vi "CMI ADS127L21 - Get Record Timestamp.vi"(8 "error in (no error)":errorcluster, 10 "Use binary mode? (False)":bool, 11 "session in":T1 {"channels"."Channel" min=1 max=8 step=1}) -> (0 "error out":errorcluster, 2 "timestamp [s]":ext, 3 "session out":T1 {"channels"."Channel" min=1 max=8 step=1})   [LabVIEW 2020]
doc: "Get timestamp of last record. USe of binary mode will transfer timestamp as int64 and then it is divided by sampling rate. This should overcome limited resolution of float64."
uses:
  CMI ADS127L21 - Session.ctl
  CMI ADS127L21 - Record Channel.ctl
  CMI ADS127L21 - Input Range.ctl
  CMI ADS127L21 - Input Mode.ctl
  CMI ADS127L21 - Input Impedance.ctl
  CMI ADS127L21 - EXTOUT Mode.ctl
  CMI ADS127L21 - EXTOUT Polarity.ctl
  <vilib>/Instr/_visa.llb/VISA Flush IO Buffer Mask.ctl
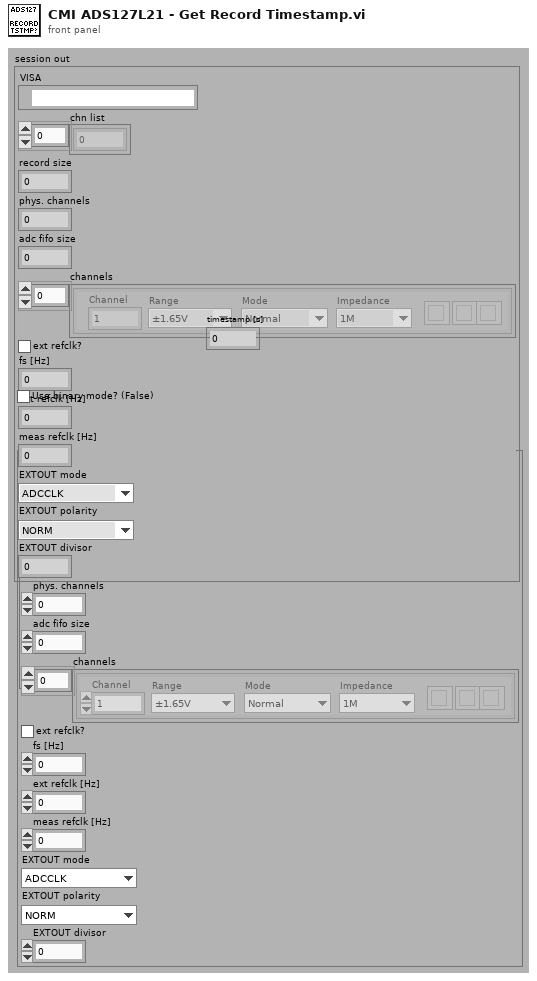
[diagram p1: front panel]
types:
  T1 = typedef "CMI ADS127L21 - Session.ctl" = cluster{"VISA":refnum<visa-resource-name>, "chn list":i32[], "record size":i32, "phys. channels":i32, "adc fifo size":i32, "channels":T2[], "ext refclk?":bool, "fs [Hz]":dbl, "ext refclk [Hz]":dbl, "meas refclk [Hz]":dbl, "EXTOUT mode":T6, "EXTOUT polarity":T7, "EXTOUT divisor":i32}
  T2 = typedef "CMI ADS127L21 - Record Channel.ctl" = cluster{"Range":T3, "Channel":i32, "Mode":T4, "Impedance":T5, "btn clr":bool, "btn up":bool, "btn down":bool}
  T3 = typedef "CMI ADS127L21 - Input Range.ctl" = enum16{"±1.65V", "±2V"}
  T4 = typedef "CMI ADS127L21 - Input Mode.ctl" = enum16{"Normal", "Inverted", "GND"}
  T5 = typedef "CMI ADS127L21 - Input Impedance.ctl" = enum16{"1M", "1k5"}
  T6 = typedef "CMI ADS127L21 - EXTOUT Mode.ctl" = enum16{"ADCCLK", "REFCLK", "SMPLCLK", "FIRST"}
  T7 = typedef "CMI ADS127L21 - EXTOUT Polarity.ctl" = enum16{"NORM", "INV"}
  T8 = typedef "VISA Flush IO Buffer Mask.ctl" = u16
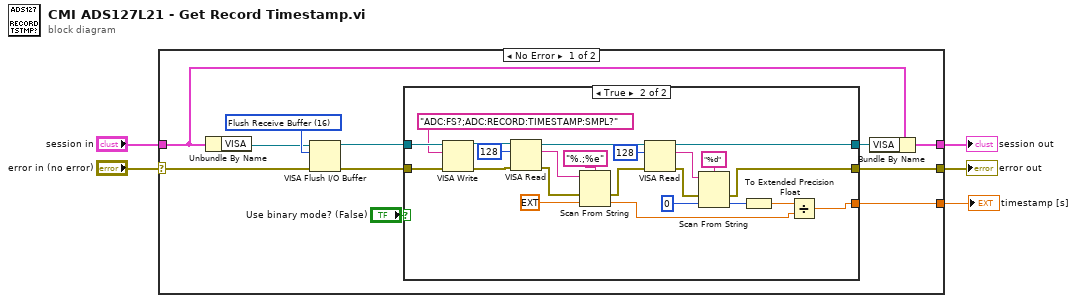
[diagram p0: block diagram]
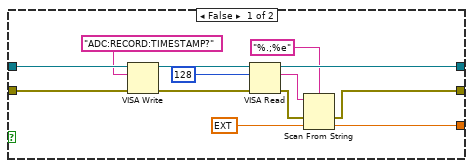
[diagram p2: hidden frame]
diagram:
  n1 = case shown="No Error" "error in (no error)" {
    selector: "error in (no error)" -> [w13 w54]
    tunnel: "session in" -> [w6 w53]
    tunnel: [w16 w53] -> w4
    tunnel: [w9 w54] -> w3
    tunnel: [w8 _] -> w1
    frame No Error {
      w15 = T8 16 items=["Flush Receive Buffer"=16, "Write Transmit Buffer to Device"=32, "Flush Receive Buffer (No I/O)"=64, "Flush Transmit Buffer"=128] ("Mask")
      n2 = Unbundle By Name(w6) -> ("VISA"=w14:refnum<visa-resource-name>)
      n3 = VISA Flush I/O Buffer(VISA resource name=w14, mask (16)=w15, error in (no error)=w13) -> (VISA resource name out=w11:refnum<visa-resource-name>, error out=w12:errorcluster)
      n4 = case shown="True" "Use binary mode? (False)" {
        tunnel: w12 -> [w29 w52]
        tunnel: w11 -> [w28 w51]
        tunnel: [w24 w49] -> w10
        tunnel: [w20 w46] -> w9
        tunnel: [w17 w41] -> w8
        frame False {
          n5 = VISA Write(VISA resource name=w28, write buffer="ADC:RECORD:TIMESTAMP?", error in (no error)=w29) -> (VISA resource name out=w25:refnum<visa-resource-name>, error out=w26:errorcluster)  [unwired: 1 out]
          n6 = VISA Read(VISA resource name=w25, byte count=u32 128, error in (no error)=w26) -> (VISA resource name out=w24:refnum<visa-resource-name>, read buffer=w21:string, error out=w22:errorcluster)  [unwired: 1 out]
          n7 = Scan From String(format string="%.;%e", input string=w21, error in=w22, default 1=ext nan) -> (error out=w20:errorcluster, output 1=w17:ext)  [unwired: 1 in, 2 out]
        }
        frame True {
          n8 = VISA Write(VISA resource name=w51, write buffer="ADC:FS?;ADC:RECORD:TIMESTAMP:SMPL?", error in (no error)=w52) -> (VISA resource name out=w33:refnum<visa-resource-name>, error out=w34:errorcluster)  [unwired: 1 out]
          n9 = VISA Read(VISA resource name=w33, byte count=u32 128, error in (no error)=w34) -> (VISA resource name out=w30:refnum<visa-resource-name>, read buffer=w38:string, error out=w37:errorcluster)  [unwired: 1 out]
          n10 = Scan From String(format string="%.;%e", input string=w38, error in=w37, default 1=ext 0.0) -> (error out=w32:errorcluster, output 1=w31:ext)  [unwired: 1 in, 2 out]
          n11 = VISA Read(VISA resource name=w30, byte count=u32 128, error in (no error)=w32) -> (VISA resource name out=w49:refnum<visa-resource-name>, read buffer=w47:string, error out=w48:errorcluster)  [unwired: 1 out]
          n12 = Scan From String(format string="%d", input string=w47, error in=w48, default 1=i64 0) -> (error out=w46:errorcluster, output 1=w43:i64)  [unwired: 1 in, 2 out]
          n13 = To Extended Precision Float(1:w43) -> (0:w42:ext)
          n14 = Divide(x=w42, y=w31) -> (x/y=w41:ext)
        }
      }
      n15 = Bundle By Name(cluster=w6, "VISA"=w10) -> (w16:T1)
    }
    frame Error {
    }
  }
  "error out" <- w3
  "session out" <- w4
  "timestamp [s]" <- w1
